vi "_Check_License.vi"(8 "error in (no error)":errorcluster) -> (0 "error out":errorcluster, 2 "License status":T1(ring))   [LabVIEW 2019, in "PG_LIB.lvlib" / "Postgres Connector.lvclass"]
doc: "Verify the licence of the lvlib."
uses:
  Postgres Connector.lvclass
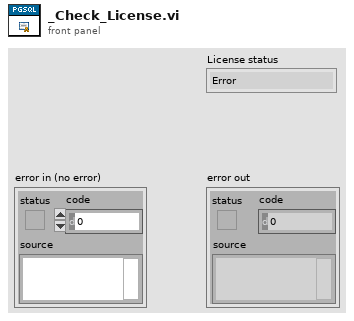
[diagram p1: front panel]
types:
  T1 = enum16{"Error", "Activated", "Evaluation", "Unlicensed"}
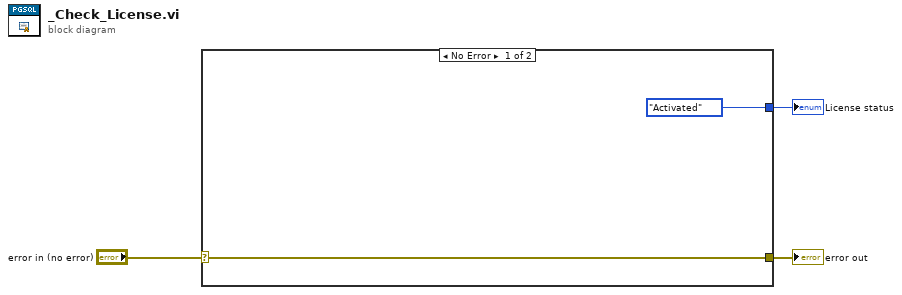
[diagram p0: block diagram]
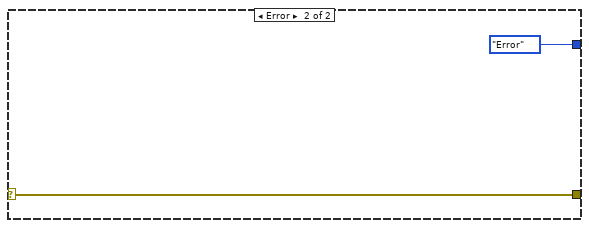
[diagram p2: hidden frame]
diagram:
  n1 = case shown="No Error" "error in (no error)" {
    selector: "error in (no error)" -> [w5 w7]
    tunnel: [w5 w7] -> w3
    tunnel: [T1."Activated" ("License status") T1."Error" ("License status")] -> w1
    frame No Error {
    }
    frame Error {
    }
  }
  "License status" <- w1
  "error out" <- w3
